vi "RSZVB Complete Noise Figure Calibration.vi"(8 "error in (no error)":errorcluster {"code" format="%.0x"}, 10 "Channel (1)":i32=1, 11 "VISA session":refnum<visa-resource-name>) -> (0 "error out":errorcluster {"code" format="%.0x"}, 3 "dup VISA session":refnum<visa-resource-name>)   [LabVIEW 2011]
doc: "This VI completes a noise figure calibration, storing and applying the acquired data\n\nNote(s):\n\n(1) This VI is available only with option R&S ZVAB-K30.\n\nRemote-control command(s):\n[SENSe<Ch>:]CORRection:COLLect:NFIGure:SAVE"
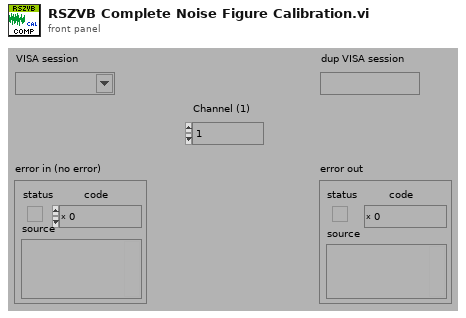
[diagram p1: front panel]
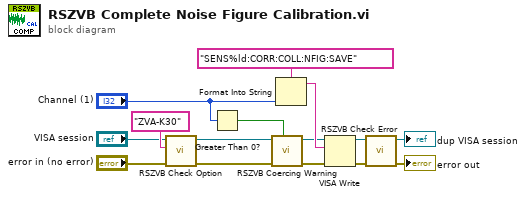
[diagram p0: block diagram]
diagram:
  n1 = call "RSZVB Check Option.vi"("error in (no error)"="error in (no error)", "Options"="ZVA-K30", "VISA session"="VISA session") -> ("error out"=w6:errorcluster, "dup VISA session"=w7:refnum<visa-resource-name>)  [unwired: 7 in]
  n2 = Greater Than 0?(x="Channel (1)") -> (x > 0?=w15:bool)
  n3 = call "RSZVB Coercing Warning.vi"("In Range?"=w15, "error in (no error)"=w6, "VISA session"=w7) -> ("error out"=w11:errorcluster, "dup VISA session"=w10:refnum<visa-resource-name>)  [unwired: 7 in]
  n4 = Format Into String(format string="SENS%ld:CORR:COLL:NFIG:SAVE", "Channel (1)") -> (resulting string=w12:string)  [unwired: 2 in, 1 out]
  n5 = VISA Write(VISA resource name=w10, write buffer=w12, error in (no error)=w11) -> (VISA resource name out=w13:refnum<visa-resource-name>, error out=w14:errorcluster)  [unwired: 1 out]
  n6 = call "RSZVB Check Error.vi"("error in (no error)"=w14, "VISA session"=w13) -> ("error out"=→"error out":errorcluster, "dup VISA session"=→"dup VISA session":refnum<visa-resource-name>)  [unwired: 8 in]
